vi "Simple Example.vi"() -> ()   [LabVIEW 2024]
uses:
  <vilib>/Analysis/Matrix/Datatypes/RealMatrix.ctl
  <vilib>/Analysis/baseanly.llb/Real A x B.vi
  <vilib>/Analysis/Matrix/NI_Matrix.lvlib
  <vilib>/Analysis/NI_AALBase.lvlib
panel:
  out "3D Picture":refnum<vi>(3d-picture)
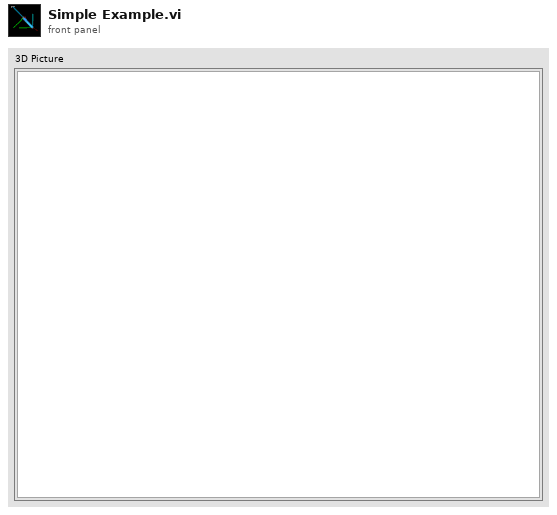
[diagram p1: front panel]
types:
  T1 = typedef "NI_Matrix.lvlib/RealMatrix.ctl" = dbl[][]
  T2 = cluster{"Line width":sgl, "Line Color":u32, "Axes?":bool}
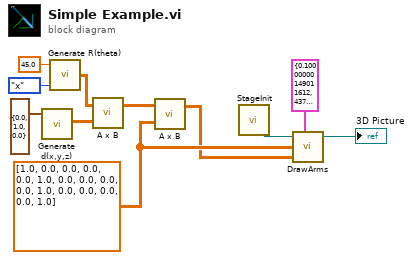
[diagram p0: block diagram]
diagram:
  w6 = T1 [[1.0, 0.0, 0.0, 0.0], [0.0, 1.0, 0.0, 0.0], [0.0, 0.0, 1.0, 0.0], [0.0, 0.0, 0.0, 1.0]] ("Start")
  n1 = call <userlib>:"Generate d(x,y,z).vi"("Translation"=cluster{"X":dbl, "Y":dbl, "Z":dbl} {"X"=0.0, "Y"=1.0, "Z"=0.0}) -> ("Transformation Matrix"=w1:T1)  [unwired: 2 in]
  n2 = call <userlib>:"Generate R(theta).vi"("Axis"=enum16{"x", "y", "z"}."x", "Angle (degrees)"=45.0) -> ("Transformation Matrix"=w2:T1)  [unwired: 1 in]
  n3 = call-poly <vilib>:"A x B.vi"("B"=w1, "A"=w2) -> ("A x B"=w3:T1)  [unwired: 1 out]
  n4 = call-poly <vilib>:"A x B.vi"("B"=w6, "A"=w3) -> ("A x B"=w5:T1)  [unwired: 1 out]
  n5 = call <userlib>:"StageInit.vi"() -> ("Stage out"=w11:refnum<vi>)  [unwired: 4 in, 1 out]
  n6 = call <userlib>:"DrawArms.vi"("Stage in"=w11, "Params"=T2 {"Line width"=0.1, "Line Color"=4376575, "Axes?"=TRUE}, "Start"=w6, "End"=w5) -> ("Stage out"=→"3D Picture":refnum<vi>)  [unwired: 2 in, 1 out]
